vi "Lake Shore 336 Write Curve.vi"(0 "VISA resource name":refnum<visa-resource-name>) -> ()   [LabVIEW 2012]
doc: "This example VI demonstrates the proper use of the Configure Curve Header and Configure Curve Point VIs. It allows the user to write a curve header, a curve point, of both."
uses:
  <instrlib>/Lake Shore 336/Lake Shore 336.lvlib
panel:
  in  "Temperature Value (0.0000)":dbl format="%.4f"
  in  "Index (1)":dbl=1.0
  in  "Units Value (0.00000)":dbl format="%.5f"
  in  "Coefficient (1:Negative)":u16(ring)=1 items=["Negative"=1, "Positive"=2]
  in  "Curve Serial Number (\"\")":string
  in  "Curve (21)":dbl=21.0
  in  "Curve Name (\"\")":string
  in  "Limit Value (375.000)":dbl=375.0 format="%.3f"
  in  "Curve Data Format (1:mV/K)":u16(ring)=1 items=["mV/K"=1, "V/K"=2, "Ohms/K"=3, "Log Ohms/K"=4]
  in  "Configure Curve Point\n (0: Configure)":u16(ring) items=["Configure", "Don't Configure"]
  in  "Configure Curve Header (0: Configure)":u16(ring) items=["Configure", "Don't Configure "]
  in  "Serial Configuration":T1={"Baud Rate"=57600, "Parity"=1, "Data Bits"=7, "Stop Bits"=10, "Flow Control"=0} {"Flow Control" items=["None", "XON/XOFF", "RTS/CTS", "XON/XOFF & RTS/CTS", "DTR/DSR", "XON/XOFF & DTR/DSR"]; "Stop Bits" items=["1.0"=10, "1.5"=15, "2.0"=20]; "Data Bits" items=["7"=7, "8"=8]; "Parity" items=["None", "Odd", "Even", "Mark", "Space"]; "Baud Rate" items=["300"=300, "600"=600, "1200"=1200, "2400"=2400, "4800"=4800, "9600"=9600, "19200"=19200, "38400"=38400, "57600"=57600]}
  # "(c) 2009 Lake Shore Cryotronics Inc.  ALL RIGHTS RESERVED."
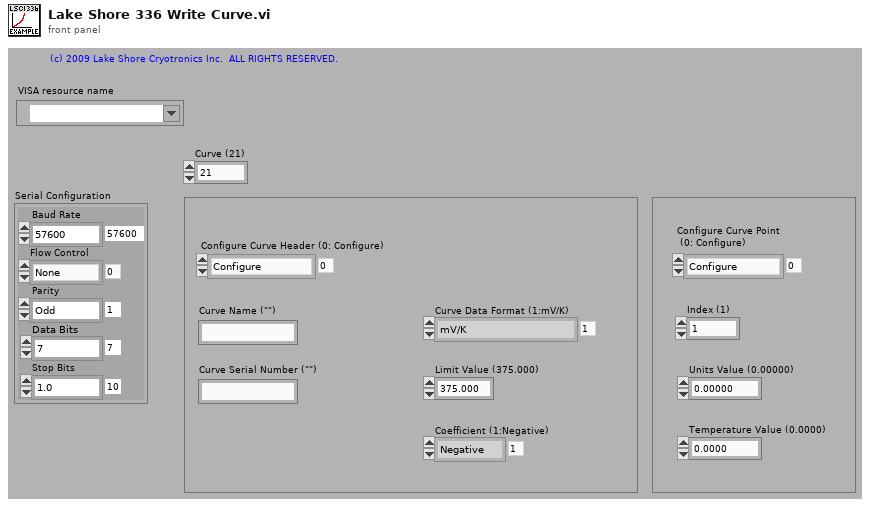
[diagram p1: front panel]
types:
  T1 = cluster{"Baud Rate":u32, "Parity":u16, "Data Bits":u16, "Stop Bits":u16, "Flow Control":u16}
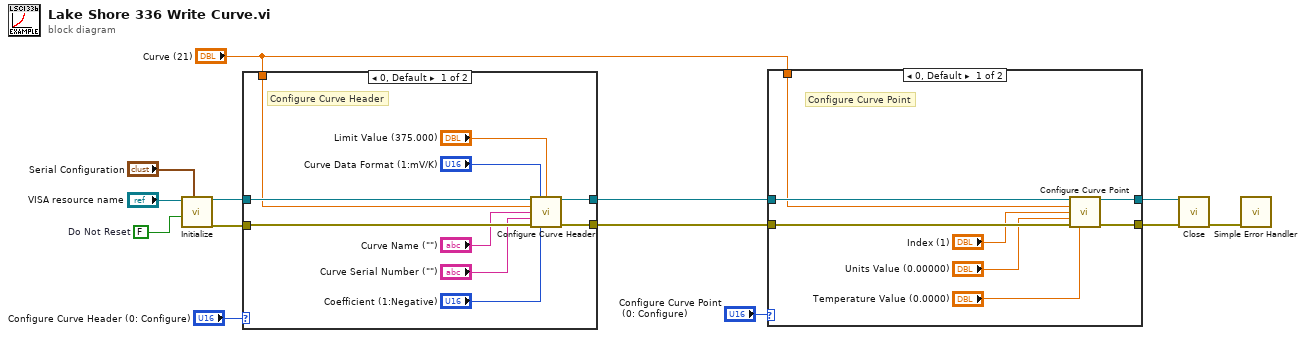
[diagram p0: block diagram]
diagram:
  w11 = FALSE  # Do Not Reset
  n1 = call <instrlib>:"Initialize.vi"("Serial Configuration"="Serial Configuration", "Reset (True)"=w11, "VISA resource name"="VISA resource name") -> ("error out"=w6:errorcluster, "VISA resource name out"=w7:refnum<visa-resource-name>)  [unwired: 7 in]
  n2 = case shown="0, Default" "Configure Curve Header (0: Configure)" {
    tunnel: w7 -> [w23 w25]
    tunnel: w6 -> [w22 w24]
    tunnel: [w21 w25] -> w5
    tunnel: [w20 w24] -> w4
    tunnel: "Curve (21)" -> [w19 _]
    frame 0, Default {
      # "Configure Curve Header"
      n3 = call <instrlib>:"Configure Curve Header.vi"("VISA resource name"=w23, "Curve Data Format (1:mV/K)"="Curve Data Format (1:mV/K)", "Limit Value (375.000)"="Limit Value (375.000)", "Curve (21)"=w19, "Curve Name (\"\")"="Curve Name (\"\")", "Curve Serial Number (\"\")"="Curve Serial Number (\"\")", "error in (no error)"=w22, "Coefficient (1:Negative)"="Coefficient (1:Negative)") -> ("VISA resource name out"=w21:refnum<visa-resource-name>, "error out"=w20:errorcluster)  [unwired: 6 in]
    }
    frame 1 {
      # "Do Not Configure Curve Header"
    }
  }
  n4 = case shown="0, Default" "Configure Curve Point\n (0: Configure)" {
    tunnel: w5 -> [w32 w35]
    tunnel: w4 -> [w33 w34]
    tunnel: [w31 w35] -> w3
    tunnel: [w30 w34] -> w2
    tunnel: "Curve (21)" -> [w29 _]
    frame 0, Default {
      # "Configure Curve Point"
      n5 = call <instrlib>:"Configure Curve Point.vi"("VISA resource name"=w32, "Curve (21)"=w29, "Index (1)"="Index (1)", "Units Value (0.00000)"="Units Value (0.00000)", "error in (no error)"=w33, "Temperature Value (0.0000)"="Temperature Value (0.0000)") -> ("VISA resource name out"=w31:refnum<visa-resource-name>, "error out"=w30:errorcluster)  [unwired: 8 in]
    }
    frame 1 {
      # "Do Not Configure Curve Point"
    }
  }
  n6 = call <instrlib>:"Close.vi"("error in (no error)"=w2, "VISA resource name"=w3) -> ("error out"=w12:errorcluster)  [unwired: 9 in]
  n7 = call <vilib>:"Simple Error Handler.vi"("error in (no error)"=w12) -> ()  [unwired: 4 in, 5 out]
